vi "Initialize Raw XNET Frame.vi"(10 "Data":u8[](array[numeric])=[0, 0, 0, 0, 0, 0, 0, 0], 11 "identifier":u32) -> (3 "Raw Frame":u8[](array[numeric]))   [LabVIEW 2013, in "Diagnostics Addon Engine.lvlib"]
uses:
  Diagnostics Addon Engine.lvlib
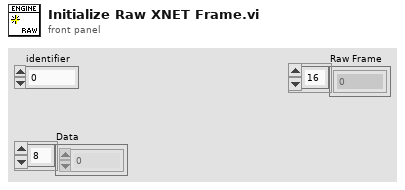
[diagram p1: front panel]
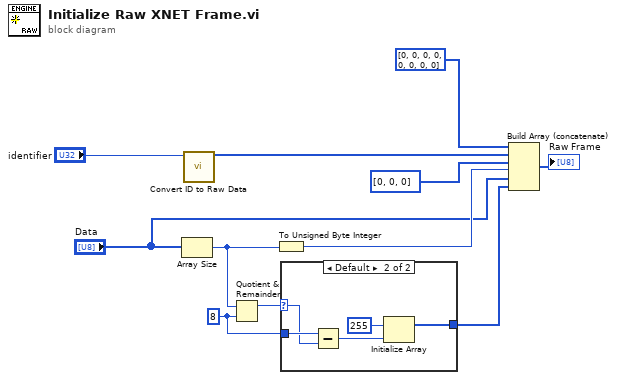
[diagram p0: block diagram]
diagram:
  w3 = 8 ("y")
  n1 = Array Size(array="Data") -> (size(s)=w4:i32)
  n2 = call "Convert ID to Raw Data.vi"("identifier"="identifier") -> ("Data"=w10:u8[])  [unwired: 10 in]
  n3 = Quotient & Remainder(x=w4, y=w3) -> (x-y*floor(x/y)=w1:i32)  [unwired: 1 out]
  n4 = To Unsigned Byte Integer(number=w4) -> (unsigned 8bit integer=w7:u8)
  n5 = case shown="Default" w1 {
    selector: w1 -> [_ w12]
    tunnel: w3 -> [_ w16]
    tunnel: [_ w13] -> w2
    frame 0 {
    }
    frame Default {
      n6 = Subtract(x=w16, y=w12) -> (x-y=w15:i32)
      n7 = Initialize Array(u8 255, w15) -> (w13:u8[])
    }
  }
  n8 = Build Array (concatenate)(u8[] [0, 0, 0, 0, 0, 0, 0, 0], w10, u8[] [0, 0, 0], w7, "Data", w2) -> (→"Raw Frame":u8[])
